vi "Align Traces to Zero.vi"(0 "Data Input":T2(array[cluster]) {"Data Channels" format="%.2f"}, 4 "Y Level":dbl format="%.2f", 5 "X Level":dbl format="%.2f", 9 "Channels / Subject (in)":T1(array[cluster])=[[{"Start"=0, "End"=1000000, "Offset"=0.0, "Deleted"=FALSE}]] {"Offset" format="%.2f"}) -> (11 "Channels / Subject (out)":T1(array[cluster])=[[{"Start"=0, "End"=1000000, "Offset"=0.0, "Deleted"=FALSE}]] {"Offset" format="%.2f"})   [LabVIEW 2016, in "impulse functions.lvlib"]
uses:
  impulse functions.lvlib
panel:
  # "Copyright Americo A. Migliaccio (c) 2002 All Rights Reserved by Author"
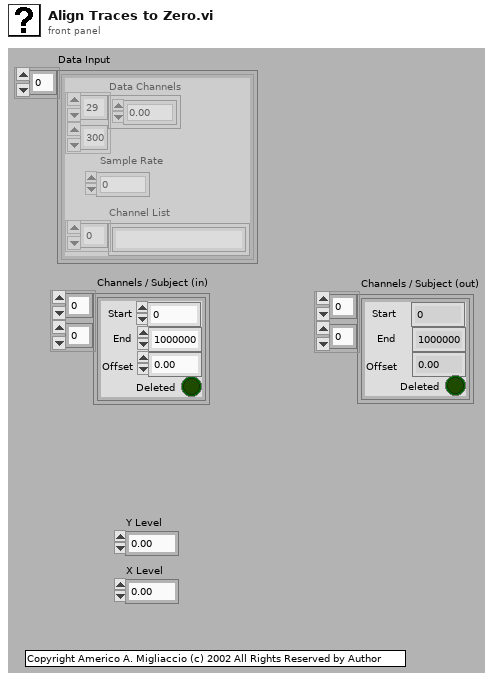
[diagram p1: front panel]
types:
  T1 = cluster{"Start":i32, "End":i32, "Offset":dbl, "Deleted":bool}[][]
  T2 = cluster{"Data Channels":dbl[][], "Sample Rate":i32, "Channel List":string[]}[]
  T3 = cluster{"Start":i32, "End":i32, "Offset":dbl, "Deleted":bool}
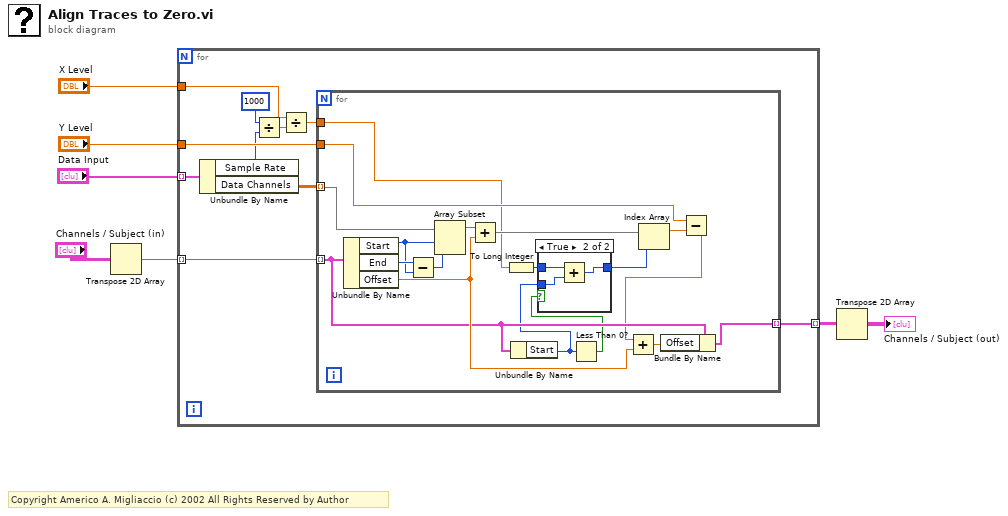
[diagram p0: block diagram]
diagram:
  # "Copyright Americo A. Migliaccio (c) 2002 All Rights Reserved by Author"
  n1 = Transpose 2D Array(2D array="Channels / Subject (in)") -> (transposed array=w2:T1)
  n2 = for {
    tunnel: "Y Level" -> [w17]
    tunnel: "X Level" -> [w12]
    tunnel: "Data Input" -> [w16] mode=indexing
    tunnel: w2 -> [w14] mode=indexing
    tunnel: [w13] -> w3 mode=indexing
    n3 = Unbundle By Name(w16) -> ("Sample Rate"=w11:i32, "Data Channels"=w15:dbl[][])
    n4 = Divide(x=1000, y=w11) -> (x/y=w8:dbl)
    n5 = Divide(x=w12, y=w8) -> (x/y=w9:dbl)
    n6 = for {
      tunnel: w17 -> [w35]
      tunnel: w15 -> [w26] mode=indexing
      tunnel: w14 -> [w25] mode=indexing
      tunnel: [w29] -> w13 mode=indexing
      tunnel: w9 -> [w28]
      n7 = Unbundle By Name(w25) -> ("Start"=w31:i32, "End"=w32:i32, "Offset"=w27:dbl)
      n8 = Subtract(x=w32, y=w31) -> (x-y=w30:i32)
      n9 = Array Subset(array=w26, index=w31, length=w30) -> (w34:dbl[])
      n10 = Add(x=w34, y=w27) -> (x+y=w33:dbl[])
      n11 = To Long Integer(number=w28) -> (32bit integer=w23:i32)
      n12 = Unbundle By Name(w25) -> ("Start"=w18:i32)
      n13 = Less Than 0?(x=w18) -> (x < 0?=w24:bool)
      n14 = case shown="True" w24 {
        tunnel: w23 -> [w36 w39]
        tunnel: [w36 w37] -> w22
        tunnel: w18 -> [_ w38]
        frame False {
        }
        frame True {
          n15 = Add(x=w39, y=w38) -> (x+y=w37:i32)
        }
      }
      n16 = Index Array(array=w33, index=w22) -> (element=w21:dbl)
      n17 = Subtract(x=w35, y=w21) -> (x-y=w19:dbl)
      n18 = Add(x=w19, y=w27) -> (x+y=w20:dbl)
      n19 = Bundle By Name(cluster=w25, "Offset"=w20) -> (w29:T3)
    }
  }
  n20 = Transpose 2D Array(2D array=w3) -> (transposed array=→"Channels / Subject (out)":T1)
